vi "DefBallOrientSkill.vi"(8 "error in (no error)":errorcluster, 9 "Robot":refnum<class "Robot.lvclass">, 10 "Game":refnum<class "Game.lvclass">, 11 "DefBallOrientSkill in":refnum<class "DefBallOrientSkill.lvclass">) -> (0 "error out":errorcluster, 2 "Robot out":refnum<class "Robot.lvclass">, 3 "DefBallOrientSkill out":refnum<class "DefBallOrientSkill.lvclass">)   [LabVIEW 2018, in "DefBallOrientSkill.lvclass"]
uses:
  DefBallOrientSkill.lvclass
  Game_class/Game.lvclass
  Robot_class/Robot.lvclass
  C:/Users/Ronaldo/Desktop/Phoenix/SSL_AI/Object_class/Object.lvclass
  Game_class/Game.lvclass/Game.ctl
  Object_class/Object.lvclass/Object.ctl
  Robot_class/Robot.lvclass/Robot.ctl
  Game_class/Read BallRef.vi
  Object_class/Read x.vi
  Object_class/Read y.vi
  Game_class/Read FieldRef.vi
  Game_class/Read Utilities.lvclass.vi
  Robot_class/Read orientation.vi
  Robot_class/Write dest_x.vi
  Robot_class/Write dest_y.vi
  Robot_class/Write dest_orientation.vi
  Ball_class/Ball.lvclass
  Field_class/Field.lvclass
  Utilities_class/Utilities.lvclass
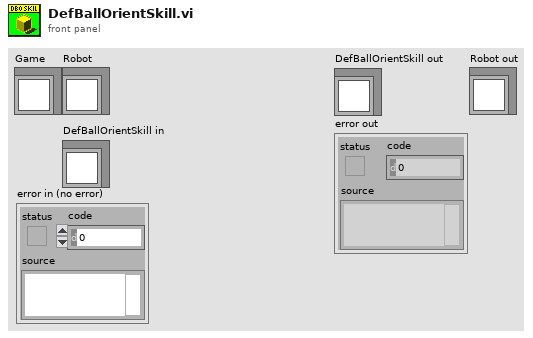
[diagram p1: front panel]
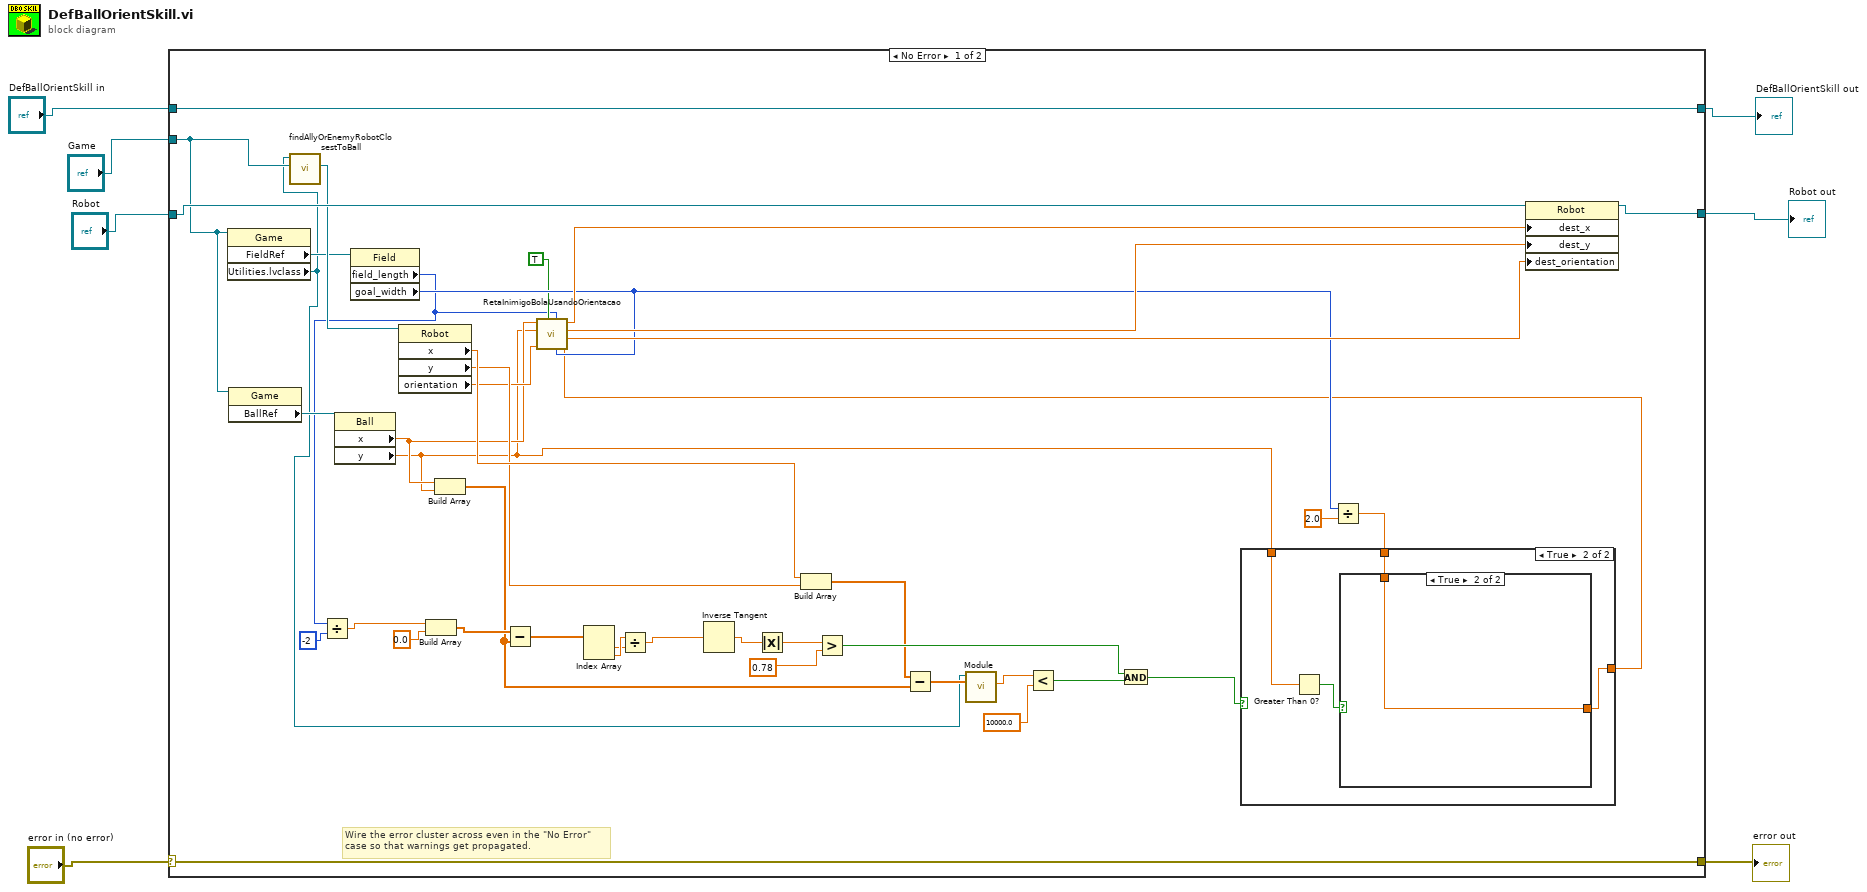
[diagram p0: block diagram]
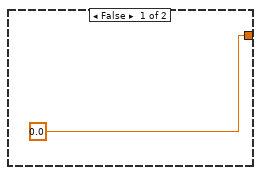
[diagram p2: hidden frame]
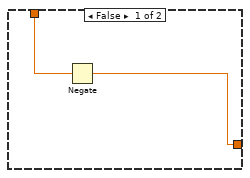
[diagram p3: hidden frame]
diagram:
  n1 = case shown="No Error" "error in (no error)" {
    selector: "error in (no error)" -> [w48 w59]
    tunnel: [w48 w59] -> w2
    tunnel: [w49 w58] -> w6
    tunnel: "DefBallOrientSkill in" -> [w49 w58]
    tunnel: "Robot" -> [w47 _]
    tunnel: "Game" -> [w45 _]
    tunnel: [w19 _] -> w1
    frame No Error {
      # "Wire the error cluster across even in the \"No Error\"\ncase so that warnings get propagated."
      n2 = property class="Game"(reference=w45) -> ("FieldRef"=w43:refnum<class "Field.lvclass">, "Utilities.lvclass"=w8:refnum<class "Utilities.lvclass">)  [unwired: 1 in, 2 out]
      n3 = property class="Game"(reference=w45) -> ("BallRef"=w44:refnum<class "Ball.lvclass">)  [unwired: 1 in, 2 out]
      n4 = call "findAllyOrEnemyRobotClosestToBall.vi"("Game"=w45, "Utilities in"=w8) -> ("Robot"=w46:refnum<class "Robot.lvclass">)  [unwired: 6 in, 3 out]
      n5 = property class="Ball"(reference=w44) -> ("x"=w12:dbl, "y"=w11:dbl)  [unwired: 1 in, 2 out]
      n6 = property class="Field"(reference=w43) -> ("field_length"=w9:i32, "goal_width"=w15:i32)  [unwired: 1 in, 2 out]
      n7 = Divide(x=w9, y=-2) -> (x/y=w35:dbl)
      n8 = property class="Robot"(reference=w46) -> ("x"=w23:dbl, "y"=w22:dbl, "orientation"=w13:dbl)  [unwired: 1 in, 2 out]
      n9 = Build Array(w35, 0.0 ("element")) -> (w38:dbl[])
      n10 = Build Array(w12, w11) -> (w20:dbl[])
      n11 = Subtract(x=w38, y=w20) -> (x-y=w37:dbl[])
      n12 = Index Array(array=w37) -> (element #1=w33:dbl, element #2=w34:dbl)  [unwired: 2 in]
      n13 = Divide(x=w34, y=w33) -> (x/y=w32:dbl)
      n14 = Inverse Tangent(1:w32) -> (0:w31:dbl)
      n15 = Absolute Value(x=w31) -> (abs(x)=w36:dbl)
      n16 = Build Array(w23, w22) -> (w21:dbl[])
      n17 = Greater?(x=w36, y=0.78) -> (0:w27:bool)
      n18 = Subtract(x=w21, y=w20) -> (x-y=w25:dbl[])
      n19 = call-dynamic "Module.vi"("2D vector"=w25, "Utilities in"=w8) -> ("Modulo"=w24:dbl)  [unwired: 7 in, 2 out]
      n20 = Less?(x=w24, y=10000.0) -> (x < y?=w28:bool)
      n21 = And(x=w27, y=w28) -> (x .and. y?=w26:bool)
      n22 = Divide(x=w15, y=2.0) -> (x/y=w42:dbl)
      n23 = case shown="True" w26 {
        tunnel: w42 -> [_ w53]
        tunnel: [0.0 w52] -> w14
        tunnel: w11 -> [_ w51]
        frame False {
        }
        frame True {
          n24 = Greater Than 0?(x=w51) -> (x > 0?=w54:bool)
          n25 = case shown="True" w54 {
            tunnel: w53 -> [w56 w57]
            tunnel: [w55 w57] -> w52
            frame False {
              n26 = Negate(x=w56) -> (-x=w55:dbl)
            }
            frame True {
            }
          }
        }
      }
      n27 = call "RetaInimigoBolaUsandoOrientacao.vi"("Y quina"=w14, "Goal Width"=w15, "Field length"=w9, "Meio?"=TRUE, "Orientação inimigo"=w13, "Y bola"=w11, "X bola"=w12) -> ("Orientação goleiro"=w16:dbl, "Y golerio"=w17:dbl, "X goleiro"=w18:dbl)  [unwired: 2 in]
      n28 = property class="Robot"(reference=w47, "dest_x"=w18, "dest_y"=w17, "dest_orientation"=w16) -> (reference out=w19:refnum<class "Robot.lvclass">)  [unwired: 1 in, 1 out]
    }
    frame Error {
    }
  }
  "DefBallOrientSkill out" <- w6
  "error out" <- w2
  "Robot out" <- w1
